vi "LMB_WallFollow.vi"(8 "behavior weights":i8[](array[numeric]), 9 "Follow right?":bool, 10 "Following Distance":i32, 11 "_sensorData":T1) -> (3 "Behavior Output":T3)   [LabVIEW 2012]
uses:
  NINJA Code/Tugboat/Robo_Programs/behaviorOutput_t.ctl
  NINJA Code/Tugboat/Robo_Programs/sensorData_t.ctl
  NINJA Code/Tugboat/Robo_Programs/irData_t.ctl
  <vilib>/Analysis/1siggen.llb/Ramp Pattern by Samples.vi
  <vilib>/gmath/statdist.llb/Normal PDF.vi
  <vilib>/gmath/NI_Gmath.lvlib
  <vilib>/Analysis/NI_AALBase.lvlib
panel:
  # "L\nE\nF\nT"
  # "C\nE\nN\nT\nE\nR"
  # "R\nI\nG\nH\nT"
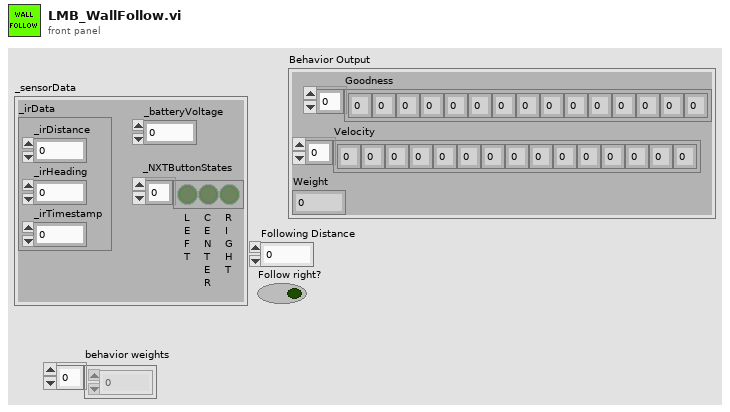
[diagram p1: front panel]
types:
  T1 = typedef "sensorData_t.ctl" = cluster{"_irData":T2, "_batteryVoltage":i32, "_NXTButtonStates":bool[]}
  T2 = typedef "irData_t.ctl" = cluster{"_irDistance":i32, "_irHeading":i32, "_irTimestamp":u32}
  T3 = typedef "behaviorOutput_t.ctl" = cluster{"Goodness":i8[], "Velocity":i8[], "Weight":i8}
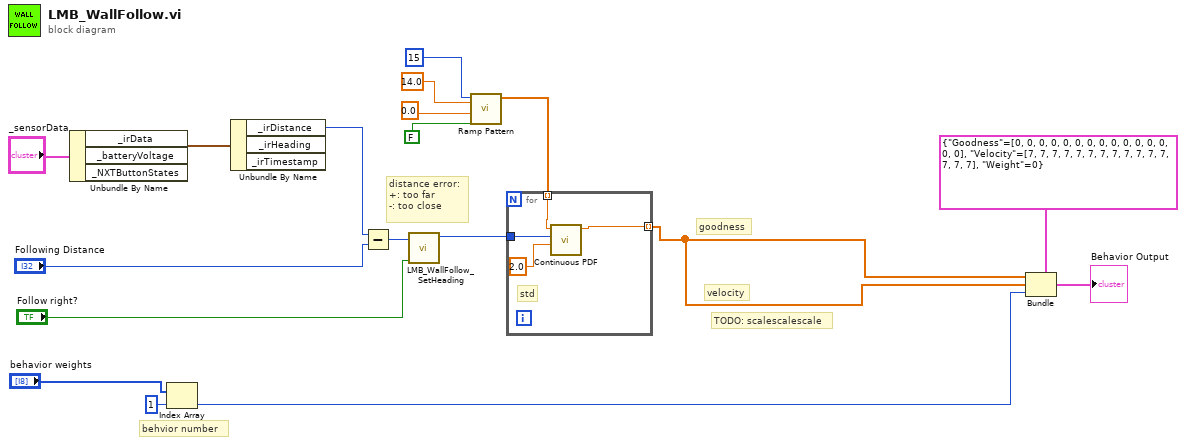
[diagram p0: block diagram]
diagram:
  # "TODO: scalescalescale"
  # "velocity"
  # "goodness"
  # "distance error: \n+: too far\n-: too close"
  # "behvior number"
  n1 = Unbundle By Name("_sensorData") -> ("_irData"=w12:T2)  [unwired: 2 out]
  n2 = Index Array(array="behavior weights", index=1) -> (element=w16:i8)
  n3 = Unbundle By Name(w12) -> ("_irDistance"=w11:i32)  [unwired: 2 out]
  n4 = Subtract(x=w11, y="Following Distance") -> (x-y=w9:i32)
  n5 = call "LMB_WallFollow_SetHeading.vi"("Follow Right?"="Follow right?", "Distance"=w9) -> ("heading"=w7:i32)  [unwired: 9 in]
  n6 = call-poly <vilib>:"Ramp Pattern.vi"("exclude end?"=FALSE, "start"=0.0, "end"=14.0, "samples"=15) -> ("Ramp Pattern"=w2:dbl[])  [unwired: 6 in, 1 out]
  n7 = for {
    tunnel: w7 -> [w22]
    tunnel: w2 -> [w20] mode=indexing
    tunnel: [w19] -> w1 mode=indexing
    # "std"
    n8 = call-poly <vilib>:"Continuous PDF.vi"("std"=2.0, "mean"=w22, "x"=w20) -> ("pdf(x)"=w19:dbl)  [unwired: 7 in, 1 out]
  }
  n9 = Bundle(cluster=T3 {"Goodness"=[0, 0, 0, 0, 0, 0, 0, 0, 0, 0, 0, 0, 0, 0, 0], "Velocity"=[7, 7, 7, 7, 7, 7, 7, 7, 7, 7, 7, 7, 7, 7, 7], "Weight"=0} ("Behavior Output"), "Goodness"=w1, "Velocity"=w1, "Weight"=w16) -> (→"Behavior Output":T3)
